vi "pulse shaping (SubVI).vi"(6 "filter parameter":dbl, 7 "IQ symbols":cdb[](array[numeric]), 9 "pulse shaping samples per symbol (16)":i32, 10 "pulse shaping filter (none)":T1(ring), 11 "modulation type":T2(ring)) -> (3 "X * Y":cdb[](array[numeric]))   [LabVIEW 2018]
uses:
  <vilib>/Analysis/2dsp.llb/1D Convolution (CDB).vi
  <vilib>/addons/Modulation/Analog/support/mod_Set Error Source.vi
  <vilib>/Analysis/2dsp.llb/Upsample (CDB).vi
  <vilib>/addons/Modulation/Digital/Support/Common/Validators/mod_Generate Filter Coefficients Validate.vi
  <vilib>/addons/Modulation/Digital/General/subVIs/mod_Generate Filter Coefficients.vi
  <vilib>/addons/Modulation/niDMT.lvlib
  <vilib>/Analysis/NI_AALPro.lvlib
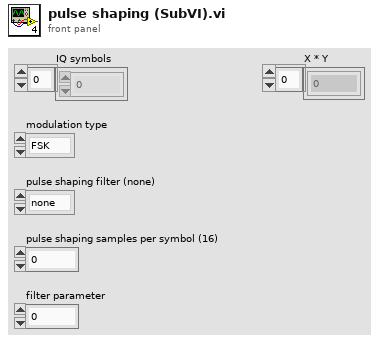
[diagram p1: front panel]
types:
  T1 = enum16{"none", "Raised Cosine", "Root Raised Cos", "Gaussian"}
  T2 = enum16{"FSK", "PSK", "QAM", "MSK", "PAM", "ASK", "CPM"}
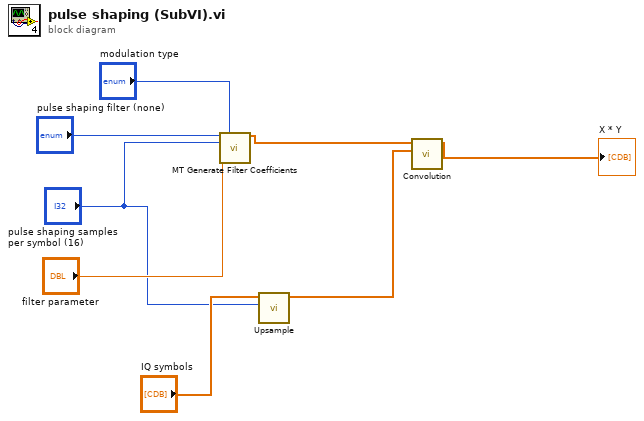
[diagram p0: block diagram]
diagram:
  n1 = call <vilib>:"MT Generate Filter Coefficients.vi"("pulse shaping filter (none)"="pulse shaping filter (none)", "modulation type"="modulation type", "pulse shaping samples per symbol (16)"="pulse shaping samples per symbol (16)", "filter parameter"="filter parameter") -> ("pulse shaping filter coefficients"=w8:dbl[])  [unwired: 9 in, 2 out]
  n2 = call-poly <vilib>:"Upsample.vi"("upsampling factor"="pulse shaping samples per symbol (16)", "X"="IQ symbols") -> ("Upsampled Array"=w7:cdb[])  [unwired: 8 in, 1 out]
  n3 = call-poly <vilib>:"Convolution.vi"("Y"=w7, "X"=w8) -> ("X * Y"=→"X * Y":cdb[])  [unwired: 8 in, 1 out]
